vi "Z_DAS - Copy.vi"(8 "下拉列表":u16(ring) items=["db", "Pa"], 9 "数组 5":dbl[][](array[numeric]), 10 "Waveform":waveform(dbl)[](array[waveform]), 11 "数组输入":dbl[][](array[numeric])) -> (1 "最小值":dbl, 2 "x-y":dbl, 3 "最大值":dbl, 4 "数组 4":dbl[][](array[numeric]), 5 "数组输出":dbl[][](array[numeric]))   [LabVIEW 2018]
uses:
  <vilib>/addons/Sound and Vibration/svt_Calibration/SVL Scale Voltage to EU (1 Ch).vi
  <vilib>/addons/_NISVFA/_Shared subVIs/Common/svc_Set SV Channel Info.vi
  <vilib>/addons/_NISVFA/_Shared subVIs/Common/svc_Set SV Channel Info (variant).vi
  <vilib>/addons/_NISVFA/_Shared subVIs/Common/SVL Set dB Reference (variant).vi
  <vilib>/addons/_NISVFA/_Shared subVIs/Common/svc_Engineering Units to Unit Label.vi
  <vilib>/addons/_NISVFA/_Shared subVIs/Common/svc_Compute Scale Factor to Convert V to EU.vi
  <vilib>/addons/_NISVFA/_Shared subVIs/Common/svc_Compute Scale Factor to Convert C to EU.vi
  <vilib>/addons/_NISVFA/_Shared subVIs/Common/svc_Set dB ref if Pascal.vi
  <vilib>/addons/_NISVFA/_Shared subVIs/Common/svc_Caller VI Returned in Error Source.vi
  <vilib>/addons/Sound and Vibration/svt_Level/SVL Running Leq Sound Level (1 Ch).vi
  <vilib>/measure/madcrms.llb/Basic Averaged DC-RMS for 1 Chan.vi
  <vilib>/measure/NI_MAPro.lvlib
  <vilib>/addons/Sound and Vibration/svt_Calibration/SoundVib_Calibration.lvlib
  <vilib>/addons/Sound and Vibration/svt_Level/SoundVib_SoundLevel.lvlib
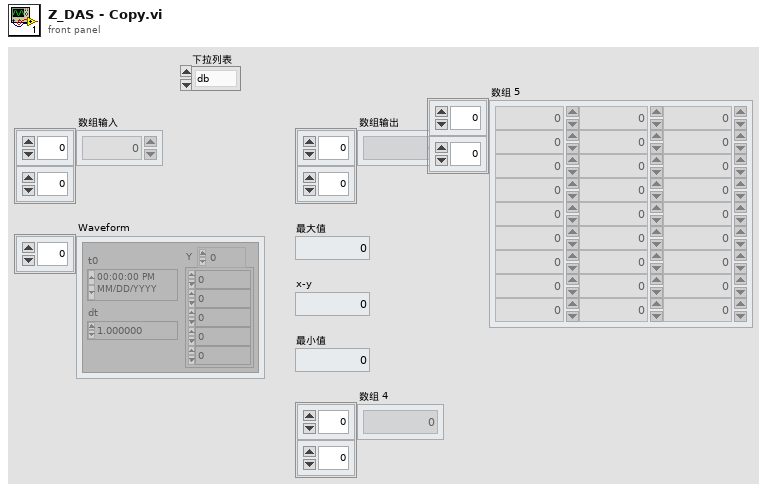
[diagram p1: front panel]
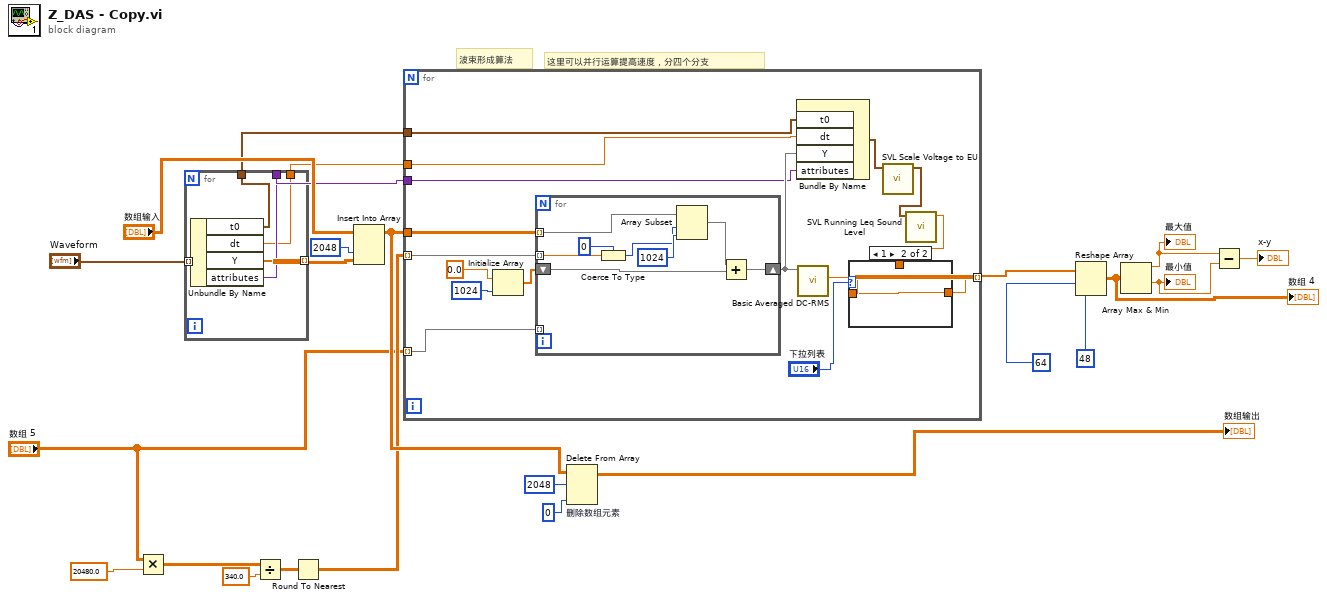
[diagram p0: block diagram]
diagram:
  # "这里可以并行运算提高速度，分四个分支"
  # "波束形成算法"
  n1 = Multiply(x="数组 5", y=20480.0) -> (x*y=w8:dbl[][])
  n2 = for {
    tunnel: "Waveform" -> [w29] mode=indexing
    tunnel: [w28] -> w20 mode=indexing
    tunnel: [w27] -> w5
    tunnel: [w26] -> w4
    tunnel: [w25] -> w3
    n3 = Unbundle By Name(w29) -> ("t0"=w26:timestamp, "dt"=w25:dbl, "Y"=w28:dbl[], "attributes"=w27:variant)
  }
  n4 = Divide(x=w8, y=340.0) -> (x/y=w7:dbl[][])
  n5 = Round To Nearest(number=w7) -> (nearest integer value=w6:dbl[][])
  n6 = Insert Into Array(array="数组输入", index (col)=2048 ("禁用的索引 (列)"), new element=w20) -> (w23:dbl[][])  [unwired: 1 in]
  n7 = for {
    tunnel: w23 -> [w45]
    tunnel: [w32] -> w11 mode=indexing
    tunnel: w6 -> [w41] mode=indexing
    tunnel: w5 -> [w39]
    tunnel: w4 -> [w36]
    tunnel: w3 -> [w35]
    tunnel: "数组 5" -> [w34] mode=indexing
    n8 = Initialize Array(0.0 ("元素"), 1024 ("维数大小")) -> (w42:dbl[])
    n9 = for {
      tunnel: w45 -> [w55] mode=indexing
      shift-right: [w52] -> w40
      shift-left: w42 -> [w53]
      tunnel: w41 -> [w51] mode=indexing
      tunnel: w34 -> [_] mode=indexing
      n10 = Coerce To Type(0:w51, 1:0 ("长度")) -> (2:w50:i32)
      n11 = Array Subset(array=w55, index=w50, length=1024 ("长度")) -> (w48:dbl[])
      n12 = Add(x=w48, y=w53) -> (x+y=w52:dbl[])
    }
    n13 = Bundle By Name("t0"=w36, "dt"=w35, "Y"=w40, "attributes"=w39) -> (w38:waveform(dbl))  [unwired: 1 in]
    n14 = call-poly <vilib>:"Basic Averaged DC-RMS.vi"("signal in"=w40) -> ("RMS value"=w31:dbl)  [unwired: 7 in, 3 out]
    n15 = call-poly <vilib>:"SVL Scale Voltage to EU.vi"("signal [V]"=w38) -> ("scaled signal [EU]"=w37:waveform(dbl))  [unwired: 8 in, 2 out]
    n16 = call-poly <vilib>:"SVL Running Leq Sound Level.vi"("scaled signal [EU]"=w37) -> ("running Leq sound level [dB EU]"=w33:dbl)  [unwired: 7 in, 3 out]
    n17 = case shown="1" "下拉列表" {
      tunnel: [w46 w47] -> w32
      tunnel: w33 -> [w46 _]
      tunnel: w31 -> [_ w47]
      frame 0, Default {
      }
      frame 1 {
      }
    }
  }
  n18 = Delete From Array "删除数组元素"(array=w23, length=2048 ("长度"), index (col)=0 ("禁用的索引 (列)")) -> (array with subset deleted=→"数组输出":dbl[][])  [unwired: 1 in, 1 out]
  n19 = Reshape Array(w11, 64 ("维数大小"), 48 ("维数大小")) -> (w15:dbl[][])
  "数组 4" <- w15
  n20 = Array Max & Min(array=w15) -> (max value=w13:dbl, min value=w12:dbl)  [unwired: 2 out]
  "最大值" <- w13
  "最小值" <- w12
  n21 = Subtract(x=w13, y=w12) -> (x-y=→"x-y":dbl)
